vi "Set Color Theme.vi"(8 "error in (no error)":errorcluster, 10 "Color Theme":enum16{"LabVIEW", "Dark", "Windows Gray"}(ring), 11 "Menu in":refnum<class "Menu.lvclass">) -> (0 "error out":errorcluster, 3 "Menu out":refnum<class "Menu.lvclass">)   [LabVIEW 2021, in "Menu.lvlib" / "Menu.lvclass"]
uses:
  Menu.lvclass
  Menu.lvclass/Menu.ctl
  Picture2D/src/Color/Color.lvclass
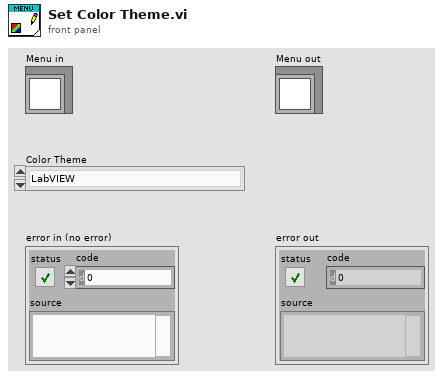
[diagram p1: front panel]
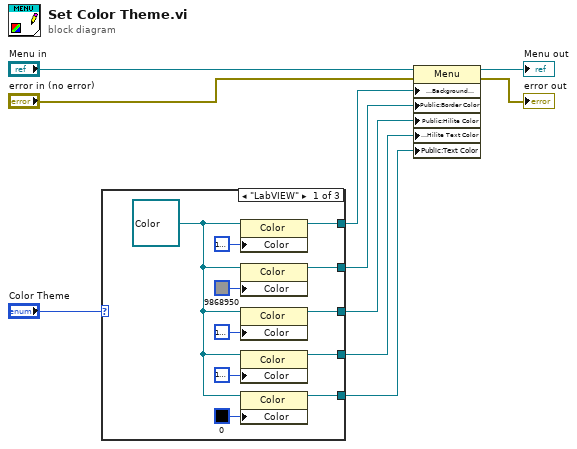
[diagram p0: block diagram]
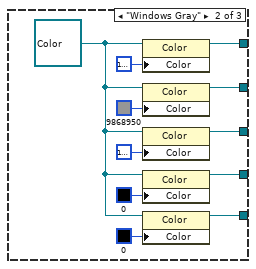
[diagram p2: hidden frame]
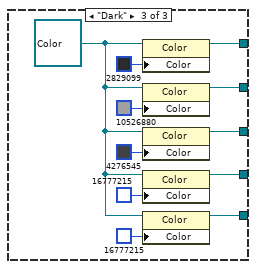
[diagram p3: hidden frame]
diagram:
  n1 = case shown="\"LabVIEW\"" "Color Theme" {
    tunnel: [w21 w32 w43] -> w4
    tunnel: [w19 w30 w41] -> w5
    tunnel: [w18 w29 w40] -> w6
    tunnel: [w17 w28 w39] -> w7
    tunnel: [w16 w27 w38] -> w8
    frame "LabVIEW" {
      w20 = refnum<class "Color.lvclass"> refnum ("Background Color")
      n2 = property class="Color"(reference=w20, "Color"=u32 16777238) -> (reference out=w21:refnum<class "Color.lvclass">)  [unwired: 1 in, 1 out]
      n3 = property class="Color"(reference=w20, "Color"=u32 9868950) -> (reference out=w19:refnum<class "Color.lvclass">)  [unwired: 1 in, 1 out]
      n4 = property class="Color"(reference=w20, "Color"=u32 16777224) -> (reference out=w18:refnum<class "Color.lvclass">)  [unwired: 1 in, 1 out]
      n5 = property class="Color"(reference=w20, "Color"=u32 16777226) -> (reference out=w17:refnum<class "Color.lvclass">)  [unwired: 1 in, 1 out]
      n6 = property class="Color"(reference=w20, "Color"=u32 0) -> (reference out=w16:refnum<class "Color.lvclass">)  [unwired: 1 in, 1 out]
    }
    frame "Windows Gray" {
      w31 = refnum<class "Color.lvclass"> refnum ("Background Color")
      n7 = property class="Color"(reference=w31, "Color"=u32 16777238) -> (reference out=w32:refnum<class "Color.lvclass">)  [unwired: 1 in, 1 out]
      n8 = property class="Color"(reference=w31, "Color"=u32 9868950) -> (reference out=w30:refnum<class "Color.lvclass">)  [unwired: 1 in, 1 out]
      n9 = property class="Color"(reference=w31, "Color"=u32 16777225) -> (reference out=w29:refnum<class "Color.lvclass">)  [unwired: 1 in, 1 out]
      n10 = property class="Color"(reference=w31, "Color"=u32 0) -> (reference out=w28:refnum<class "Color.lvclass">)  [unwired: 1 in, 1 out]
      n11 = property class="Color"(reference=w31, "Color"=u32 0) -> (reference out=w27:refnum<class "Color.lvclass">)  [unwired: 1 in, 1 out]
    }
    frame "Dark" {
      w42 = refnum<class "Color.lvclass"> refnum ("Background Color")
      n12 = property class="Color"(reference=w42, "Color"=u32 2829099) -> (reference out=w43:refnum<class "Color.lvclass">)  [unwired: 1 in, 1 out]
      n13 = property class="Color"(reference=w42, "Color"=u32 10526880) -> (reference out=w41:refnum<class "Color.lvclass">)  [unwired: 1 in, 1 out]
      n14 = property class="Color"(reference=w42, "Color"=u32 4276545) -> (reference out=w40:refnum<class "Color.lvclass">)  [unwired: 1 in, 1 out]
      n15 = property class="Color"(reference=w42, "Color"=u32 16777215) -> (reference out=w39:refnum<class "Color.lvclass">)  [unwired: 1 in, 1 out]
      n16 = property class="Color"(reference=w42, "Color"=u32 16777215) -> (reference out=w38:refnum<class "Color.lvclass">)  [unwired: 1 in, 1 out]
    }
  }
  n17 = property class="Menu"(reference="Menu in", error in="error in (no error)", "Public:Background Color"=w4, "Public:Border Color"=w5, "Public:Hilite Color"=w6, "Public:Hilite Text Color"=w7, "Public:Text Color"=w8) -> (reference out=→"Menu out":refnum<class "Menu.lvclass">, error out=→"error out":errorcluster)
